vi "Double_GeneralGearShift_WithDeadTime.vi"(6 "error In":errorcluster, 7 "ShifterRef":T1={"DevStatus"={"status"=FALSE, "code"=0, "source"=""}, "Pneumatics Control Module"=0, "Forward Solenoid Channel"=enum."Invalid", "Reverse Solenoid Channel"=enum."Invalid"}, 9 "Shift Value":T3, 10 "Right":dbl, 11 "Left":dbl) -> (0 "error out":errorcluster, 1 "Shifting":bool, 2 "Right Output":dbl, 3 "Left Output":dbl)   [LabVIEW 2016]
uses:
  <vilib>/Rock Robotics/WPI/Solenoid/WPI_SolenoidValue.ctl
  <vilib>/Rock Robotics/WPI/Solenoid/WPI_SolenoidDevRef.ctl
  <vilib>/Rock Robotics/WPI/Solenoid/WPI_SolenoidChannel.ctl
  <vilib>/Rock Robotics/WPI/ThirdParty/CanMotor/TalonSRX/WPI_CANTalonSRX_BrakeOverride.ctl
  <vilib>/Rock Robotics/WPI/Solenoid/WPI_SolenoidSetEnum.vi
panel:
  out "Right Starting Point":dbl
  out "Left Starting Point":dbl
  out "TempTimeVal":u32
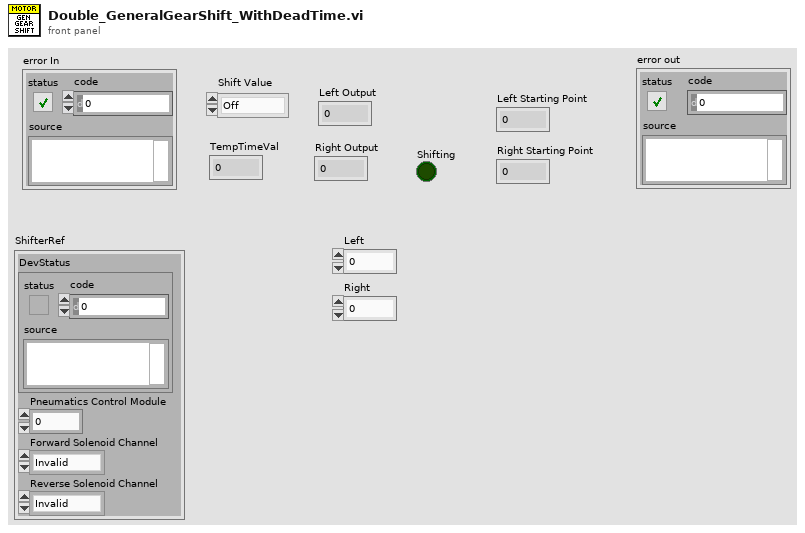
[diagram p1: front panel]
types:
  T1 = typedef "WPI_SolenoidDevRef.ctl" = cluster{"DevStatus":errorcluster, "Pneumatics Control Module":u8, "Forward Solenoid Channel":T2, "Reverse Solenoid Channel":T2}
  T2 = typedef "WPI_SolenoidChannel.ctl" = enum8{"Solenoid 0", "Solenoid 1", "Solenoid 2", "Solenoid 3", "Solenoid 4", "Solenoid 5", "Solenoid 6", "Solenoid 7", "Invalid"}
  T3 = typedef "WPI_SolenoidValue.ctl" = enum16{"Off", "On", "Forward", "Reverse"}
  T4 = typedef "WPI_MotorControlDeviceRef.ctl" = cluster{"DeviceStatus":errorcluster, "Type":T5, "PWM":cluster{"PWM Channel":T6, "DeadBand":T7}, "CAN":cluster{"Device Number":u8, "SetOutput VI Ref":variant, "GetOutput VI Ref":variant, "Enable VI Ref":variant, "Disable VI Ref":variant, "Data":variant}, "Invert":bool}
  T5 = typedef "WPI_MotorControlType.ctl" = enum16{"PWM", "CAN"}
  T6 = typedef "FPGA_DIOPWMChannel.ctl" = enum8{"PWM 0", "PWM 1", "PWM 2", "PWM 3", "PWM 4", "PWM 5", "PWM 6", "PWM 7", "PWM 8", "PWM 9", "PWM MXP 0", "PWM MXP 1", "PWM MXP 2", "PWM MXP 3", "PWM MXP 4", "PWM MXP 5", "PWM MXP 6", "PWM MXP 7", "PWM MXP 8", "PWM MXP 9", "Invalid"}
  T7 = typedef "WPI_PWMDeadband.ctl" = cluster{"Name":string, "maxPositivePwm":i32, "minPositivePwm":i32, "centerPwm":i32, "maxNegativePwm":i32, "minNegativePwm":i32, "angularRange":u16}
  T8 = typedef "WPI_CANTalonSRX_BrakeOverride.ctl" = enum8{"No Override", "Override to Coast", "Override to Brake"}
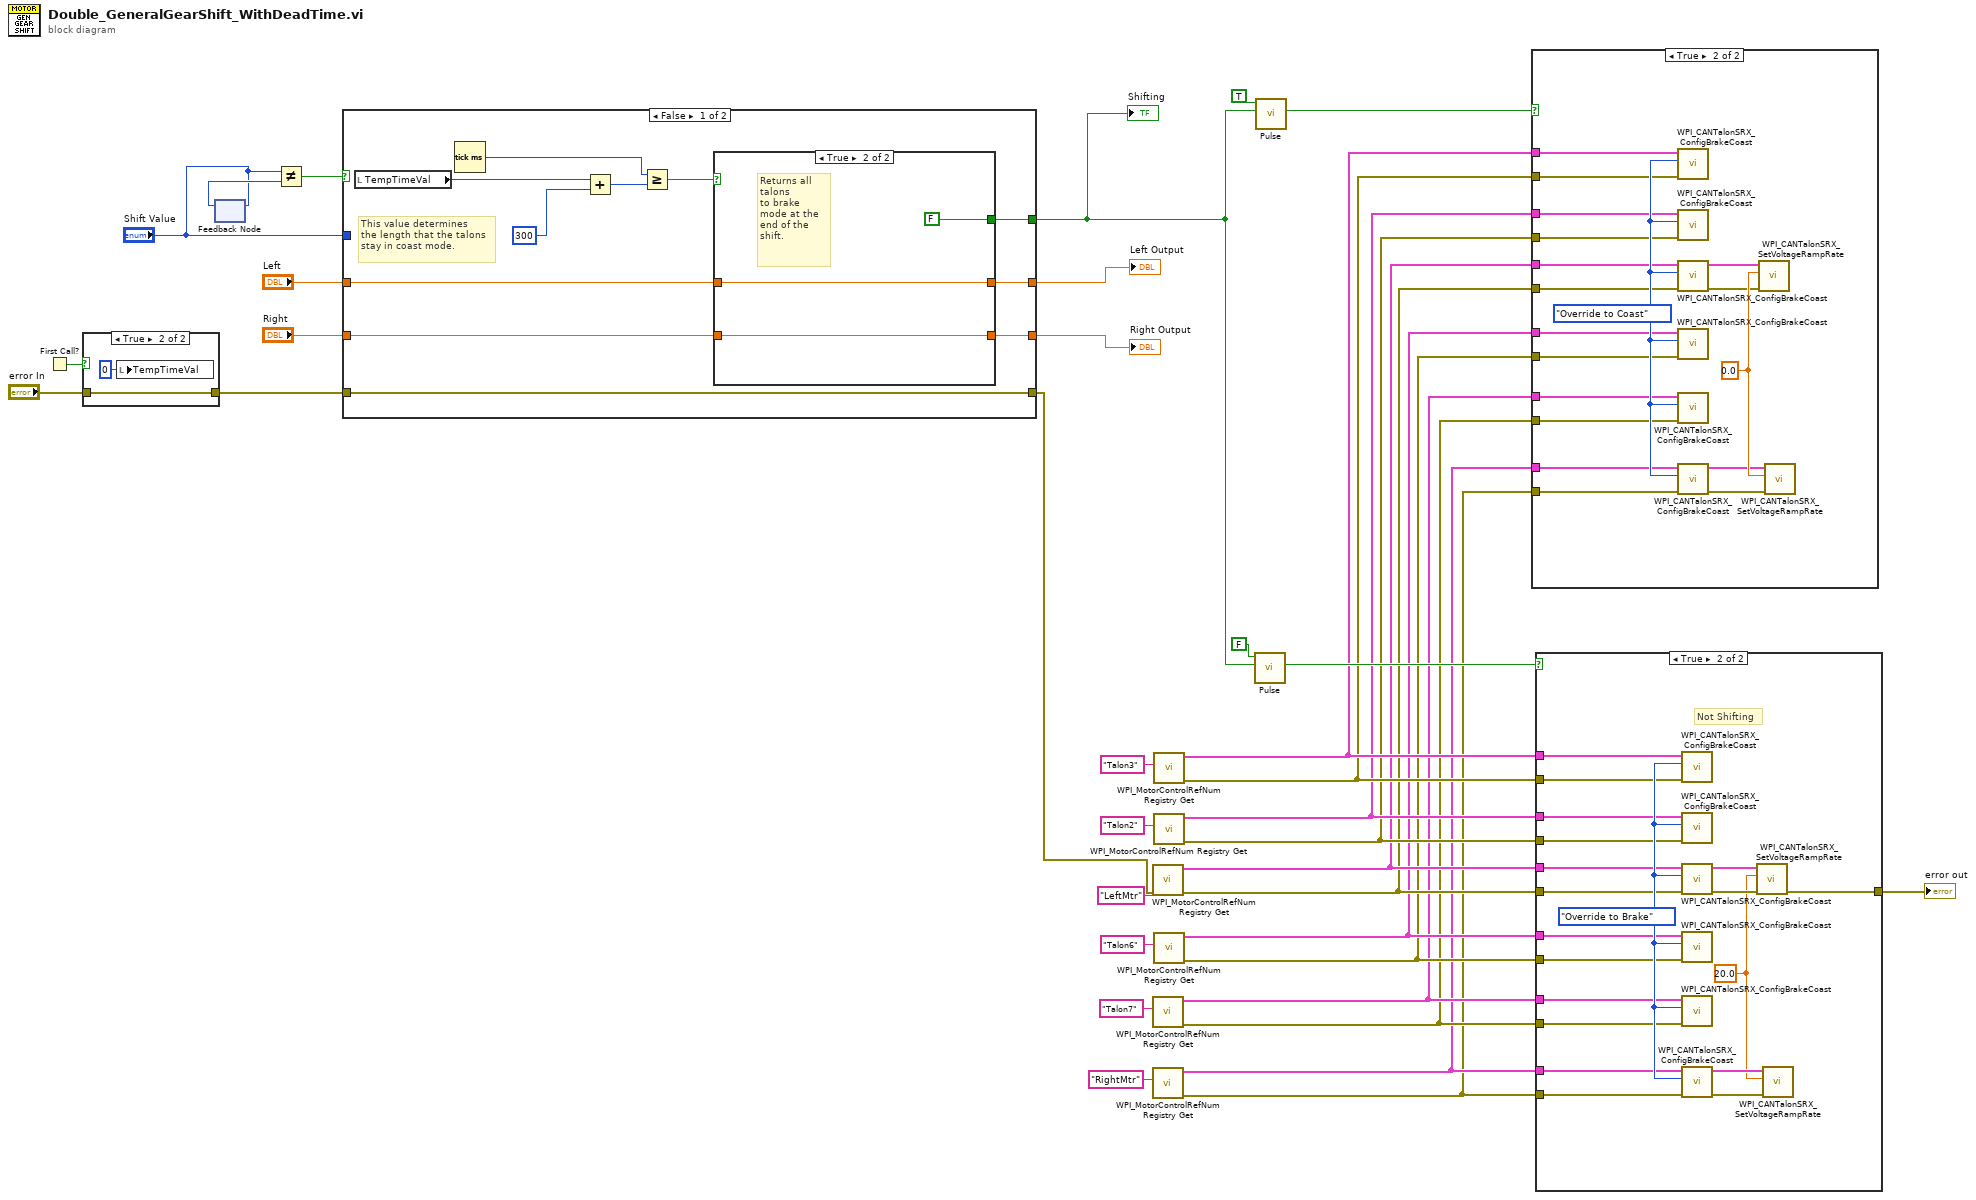
[diagram p0: block diagram]
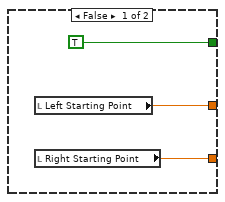
[diagram p5: hidden frame]
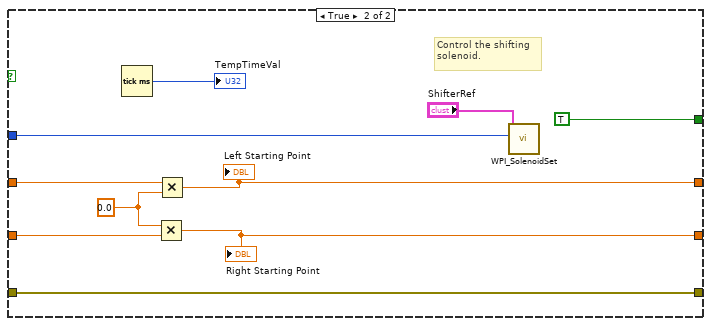
[diagram p6: hidden frame]
diagram:
  n1 = First Call?() -> (First Call?: T/F=w31:bool)
  n2 = case shown="True" w31 {
    tunnel: [w36 w37] -> w3
    tunnel: "error In" -> [w36 w37]
    frame False {
    }
    frame True {
      n3 = local write "TempTimeVal"(u32 0 ("TempTimeVal")) -> ()
    }
  }
  n4 = feedback-in #1("Shift Value") -> ()
  n5 = feedback #1() -> (w29:T3)  [unwired: 1 in]
  n6 = Not Equal?(x="Shift Value", y=w29) -> (x != y?=w28:bool)
  n7 = case shown="False" w28 {
    tunnel: [w49 w61] -> w35
    tunnel: [w48 w60] -> w34
    tunnel: "Right" -> [w47 w63]
    tunnel: "Left" -> [w46 w64]
    tunnel: [w40 TRUE] -> w23
    tunnel: "Shift Value" -> [_ w57]
    tunnel: w3 -> [w39 w56]
    tunnel: [w39 w56] -> w1
    frame False {
      # "This value determines\nthe length that the talons\nstay in coast mode."
      n8 = local read "TempTimeVal"() -> (w42:u32)
      n9 = Tick Count (ms)() -> (millisecond timer value=w44:u32)
      n10 = Add(x=w42, y=300) -> (x+y=w43:u32)
      n11 = Greater Or Equal?(x=w44, y=w43) -> (x >= y?=w45:bool)
      n12 = case shown="True" w45 {
        tunnel: [w51 w54] -> w49
        tunnel: [w52 w55] -> w48
        tunnel: w47 -> [_ w55]
        tunnel: w46 -> [_ w54]
        tunnel: [TRUE FALSE] -> w40
        frame False {
          n13 = local read "Left Starting Point"() -> (w51:dbl)
          n14 = local read "Right Starting Point"() -> (w52:dbl)
        }
        frame True {
          # "Returns all talons\nto brake mode at the\nend of the shift."
        }
      }
    }
    frame True {
      w62 = 0.0
      # "Control the shifting\nsolenoid."
      n15 = Tick Count (ms)() -> (millisecond timer value=→"TempTimeVal":u32)
      n16 = Multiply(x=w62, y=w63) -> (x*y=w60:dbl)
      "Right Starting Point" <- w60
      n17 = Multiply(x=w64, y=w62) -> (x*y=w61:dbl)
      "Left Starting Point" <- w61
      n18 = call-poly <vilib>:"WPI_SolenoidSet.vi"("Value"=w57, "SolenoidDevRef"="ShifterRef") -> ()  [unwired: 8 in, 2 out]
    }
  }
  "Left Output" <- w35
  "Right Output" <- w34
  "Shifting" <- w23
  n19 = call <vilib>:"WPI_MotorControlRefNum Registry Get.vi"("error in (no error)"=w1, "refnum name"="LeftMtr") -> ("error out"=w11:errorcluster, "MotorControlDevRef"=w12:T4)  [unwired: 8 in]
  n20 = call <vilib>:"WPI_MotorControlRefNum Registry Get.vi"("refnum name"="Talon7") -> ("error out"=w7:errorcluster, "MotorControlDevRef"=w8:T4)  [unwired: 9 in]
  n21 = call <vilib>:"WPI_MotorControlRefNum Registry Get.vi"("refnum name"="RightMtr") -> ("error out"=w5:errorcluster, "MotorControlDevRef"=w6:T4)  [unwired: 9 in]
  n22 = call <vilib>:"WPI_MotorControlRefNum Registry Get.vi"("refnum name"="Talon3") -> ("error out"=w15:errorcluster, "MotorControlDevRef"=w16:T4)  [unwired: 9 in]
  n23 = call <vilib>:"WPI_MotorControlRefNum Registry Get.vi"("refnum name"="Talon2") -> ("error out"=w13:errorcluster, "MotorControlDevRef"=w14:T4)  [unwired: 9 in]
  n24 = call <vilib>:"WPI_MotorControlRefNum Registry Get.vi"("refnum name"="Talon6") -> ("error out"=w9:errorcluster, "MotorControlDevRef"=w10:T4)  [unwired: 9 in]
  n25 = call "Pulse.vi"("Input"=w23, "Rising Edge?"=FALSE) -> ("Output"=w25:bool)  [unwired: 9 in]
  n26 = call "Pulse.vi"("Input"=w23, "Rising Edge?"=TRUE) -> ("Output"=w4:bool)  [unwired: 9 in]
  n27 = case shown="True" w4 {
    tunnel: w16 -> [_ w82]
    tunnel: w15 -> [_ w81]
    tunnel: w14 -> [_ w80]
    tunnel: w13 -> [_ w79]
    tunnel: w11 -> [_ w77]
    tunnel: w12 -> [_ w78]
    tunnel: w10 -> [_ w76]
    tunnel: w9 -> [_ w75]
    tunnel: w8 -> [_ w74]
    tunnel: w7 -> [_ w73]
    tunnel: w6 -> [_ w72]
    tunnel: w5 -> [_ w71]
    frame False {
    }
    frame True {
      w70 = 0.0 ("Throttle Ramp Rate (percent/s)")
      w83 = WPI_CANTalonSRX_BrakeOverride."Override to Coast" ("Brake / Coast Mode")
      n28 = call <vilib>:"WPI_CANTalonSRX_ConfigBrakeCoast.vi"("error in (no error)"=w81, "Brake / Coast Mode"=w83, "CAN Talon SRX Ref"=w82) -> ()  [unwired: 7 in, 2 out]
      n29 = call <vilib>:"WPI_CANTalonSRX_ConfigBrakeCoast.vi"("error in (no error)"=w79, "Brake / Coast Mode"=w83, "CAN Talon SRX Ref"=w80) -> ()  [unwired: 7 in, 2 out]
      n30 = call <vilib>:"WPI_CANTalonSRX_ConfigBrakeCoast.vi"("error in (no error)"=w77, "Brake / Coast Mode"=w83, "CAN Talon SRX Ref"=w78) -> ("error out"=w67:errorcluster, "CAN Talon SRX Ref"=w66:T4)  [unwired: 7 in]
      n31 = call <vilib>:"WPI_CANTalonSRX_ConfigBrakeCoast.vi"("error in (no error)"=w75, "Brake / Coast Mode"=w83, "CAN Talon SRX Ref"=w76) -> ()  [unwired: 7 in, 2 out]
      n32 = call <vilib>:"WPI_CANTalonSRX_ConfigBrakeCoast.vi"("error in (no error)"=w73, "Brake / Coast Mode"=w83, "CAN Talon SRX Ref"=w74) -> ()  [unwired: 7 in, 2 out]
      n33 = call <vilib>:"WPI_CANTalonSRX_ConfigBrakeCoast.vi"("error in (no error)"=w71, "Brake / Coast Mode"=w83, "CAN Talon SRX Ref"=w72) -> ("error out"=w69:errorcluster, "CAN Talon SRX Ref"=w68:T4)  [unwired: 7 in]
      n34 = call <vilib>:"WPI_CANTalonSRX_SetVoltageRampRate.vi"("error in (no error)"=w67, "Throttle Ramp Rate (percent/s)"=w70, "CAN Talon SRX Ref"=w66) -> ()  [unwired: 7 in, 2 out]
      n35 = call <vilib>:"WPI_CANTalonSRX_SetVoltageRampRate.vi"("error in (no error)"=w69, "Throttle Ramp Rate (percent/s)"=w70, "CAN Talon SRX Ref"=w68) -> ()  [unwired: 7 in, 2 out]
    }
  }
  n36 = case shown="True" w25 {
    tunnel: w16 -> [_ w102]
    tunnel: w15 -> [_ w101]
    tunnel: w14 -> [_ w100]
    tunnel: w13 -> [_ w99]
    tunnel: w11 -> [w84 w97]
    tunnel: w12 -> [_ w98]
    tunnel: w10 -> [_ w96]
    tunnel: w9 -> [_ w95]
    tunnel: w8 -> [_ w94]
    tunnel: w7 -> [_ w93]
    tunnel: w6 -> [_ w92]
    tunnel: w5 -> [_ w91]
    tunnel: [w84 w85] -> w2
    frame False {
    }
    frame True {
      w86 = 20.0 ("Throttle Ramp Rate (percent/s)")
      w103 = WPI_CANTalonSRX_BrakeOverride."Override to Brake" ("Brake / Coast Mode")
      # "Not Shifting"
      n37 = call <vilib>:"WPI_CANTalonSRX_ConfigBrakeCoast.vi"("error in (no error)"=w101, "Brake / Coast Mode"=w103, "CAN Talon SRX Ref"=w102) -> ()  [unwired: 7 in, 2 out]
      n38 = call <vilib>:"WPI_CANTalonSRX_ConfigBrakeCoast.vi"("error in (no error)"=w99, "Brake / Coast Mode"=w103, "CAN Talon SRX Ref"=w100) -> ()  [unwired: 7 in, 2 out]
      n39 = call <vilib>:"WPI_CANTalonSRX_ConfigBrakeCoast.vi"("error in (no error)"=w97, "Brake / Coast Mode"=w103, "CAN Talon SRX Ref"=w98) -> ("error out"=w87:errorcluster, "CAN Talon SRX Ref"=w88:T4)  [unwired: 7 in]
      n40 = call <vilib>:"WPI_CANTalonSRX_ConfigBrakeCoast.vi"("error in (no error)"=w95, "Brake / Coast Mode"=w103, "CAN Talon SRX Ref"=w96) -> ()  [unwired: 7 in, 2 out]
      n41 = call <vilib>:"WPI_CANTalonSRX_ConfigBrakeCoast.vi"("error in (no error)"=w93, "Brake / Coast Mode"=w103, "CAN Talon SRX Ref"=w94) -> ()  [unwired: 7 in, 2 out]
      n42 = call <vilib>:"WPI_CANTalonSRX_ConfigBrakeCoast.vi"("error in (no error)"=w91, "Brake / Coast Mode"=w103, "CAN Talon SRX Ref"=w92) -> ("error out"=w90:errorcluster, "CAN Talon SRX Ref"=w89:T4)  [unwired: 7 in]
      n43 = call <vilib>:"WPI_CANTalonSRX_SetVoltageRampRate.vi"("error in (no error)"=w87, "Throttle Ramp Rate (percent/s)"=w86, "CAN Talon SRX Ref"=w88) -> ("error out"=w85:errorcluster)  [unwired: 7 in, 1 out]
      n44 = call <vilib>:"WPI_CANTalonSRX_SetVoltageRampRate.vi"("error in (no error)"=w90, "Throttle Ramp Rate (percent/s)"=w86, "CAN Talon SRX Ref"=w89) -> ()  [unwired: 7 in, 2 out]
    }
  }
  "error out" <- w2
